vi "FPGA Top - Packet TX Only.vi"() -> ()   [LabVIEW 2017, in "My Network FPGA v1.lvlib"]
uses:
  My Network FPGA v1.lvlib
  <instrlib>/_niInstr/Network/Types/v1/MAC Address.ctl
  <instrlib>/_niInstr/Network/Types/v1/IPv4 Address.ctl
  <instrlib>/_niInstr/Network/Ethernet/MAC/CLIP/v1/Resources.ctl
  <vilib>/Platform/TimedLoop/XDataNode/timing_clust.ctl
  <vilib>/Platform/TimedLoop/XDataNode/nitl_modes.ctl
  <vilib>/Platform/TimedLoop/XDataNode/wakeup.ctl
  <vilib>/rvi/Emulation/niFpgaGetClockAttributes.vi
  <vilib>/rvi/Emulation/niFpgaSctlEmulationGetInTimedLoop.vi
  <vilib>/rvi/Emulation/niFpgaEmulationReportErrorSimple.vi
  <vilib>/rvi/DataTransferAndStorage/Container/Common/niFpgaContainerGetUniqueNameForEmu.vi
  <vilib>/rvi/DataTransferAndStorage/Container/Common/niFpgaContainerSetEmuInfo.vi
  <vilib>/rvi/eio/common/nirviEmuReportErrorAndStop.vi
  <vilib>/rvi/Emulation/niFpgaProcessEmulError.vi
  <vilib>/rvi/DataTransferAndStorage/Container/Common/niFpgaContainerExecOnDevCompGetState.vi
  <vilib>/rvi/Emulation/niFpgaEmulationIsFPGAContextNoSignature.vi
  <vilib>/rvi/errors/niFpgaSetErrorForExecOnDevCompSimple.vi
  <vilib>/rvi/FIFO/Fifo_Resource/nirvififoEmulationSetSize.vi
  <vilib>/rvi/FIFO/Fifo_Resource/nirviFifoEmulationQueueMgr.vi
  <instcachedir>/0/nirviFifoEmulationQueueMgr_E5CAEC123FF24DC58D834DCA3CDAA9B5.lvgen/nirviFifoEmulationQueueMgr_E5CAEC123FF24DC58D834DCA3CDAA9B5_003.vi
  <vilib>/rvi/FIFO/Fifo_Resource/nirvififoEmulationDetermineInputValidOut.vi
  <vilib>/rvi/FIFO/Fifo_Resource/nirvififoEmulationCreateLock.vi
  <vilib>/rvi/FIFO/Fifo_Resource/nirvififoEmulationObtainLock.vi
  <vilib>/rvi/FIFO/Fifo_Resource/nirvififoEmulationReleaseLock.vi
  <vilib>/rvi/occurrence/nirviWaitOnOccurrenceBase.vi
  <vilib>/rvi/errors/nirviReportUnexpectedCaseInternalError.vi
  <vilib>/rvi/errors/nirviReportUnexpectedCaseInternalError (U32).vi
  <vilib>/Utility/error.llb/Clear Errors.vi
  <vilib>/rvi/interface/RandomDataEmulation/niFpgaRandomDataHandleErrors.vi
  <vilib>/rvi/Emulation/niFpgaCriticalErrorInLSC.vi
  <vilib>/rvi/eio/common/nirviEmuTemplateMethod_errors.vi
  <vilib>/Platform/TimedLoop/XDataNode/XDataNode.xnode
  <vilib>/rvi/LocalResourceManager/LocalResourceManager.xnode
  <vilib>/rvi/DataTransferAndStorage/Container/XNode/niFpgaContainer.xnode
  <vilib>/rvi/FIFO/Fifo_Resource/niFpgaFifoEmulationRefIn.vi
  <vilib>/eio/EIONode/EIONode.xnode
  <instrlib>/_niInstr/Network/Ethernet/MAC/CLIP/v1/niInstr Ethernet MAC - CLIP v1.lvclass
  <instrlib>/_niInstr/Network/Ethernet/MAC/Raw Stream/v1/niInstr Ethernet MAC Raw Stream v1.lvclass
  <vilib>/Platform/TimedLoop/XDataNode/XDNodeRunTimeDep.lvlib
  <instrlib>/_niInstr/Network/IPv4/UDP/FPGA/v1/niInstr IPv4 UDP FPGA v1.lvlib
  <instrlib>/_niInstr/Network/Types/v1/niInstr Network Types v1.lvlib
panel:
  in  "enable tx":bool=TRUE
  in  "max payload per frame":u16=1472
  in  "send packet":bool
  in  "udp payload length":u16=1024
  out "aBlockLockPort0":bool
  out "aBlockLockPort1":bool
  out "mgtrefclks_locked":bool
  out "mgtrefclks_valid":bool
  out "posc_complete":bool
  out "sPort0_Power_Good":bool
  out "sPort1_Power_Good":bool
  out "signal_detect_Port0":bool
  out "signal_detect_Port1":bool
  in  "UDP destination port":u16=35311
  in  "MAC destination address":T1=[255, 255, 255, 255, 255, 255] format="%.0x"
  in  "IPv4 destination address":T2=[255, 255, 255, 255]
  in  "UDP source port":u16
  in  "IPv4 source address":T2=[0, 0, 0, 0]
  in  "MAC source address":T1=[0, 128, 47, 0, 0, 1] format="%.0x"
  # "License Note\n\nThis example makes use of code under the LGPLv2 license in the Socketed CLIP to support 10 Gigabit Ethernet.  You may find the source and build instructions for this component in the CLIP directory."
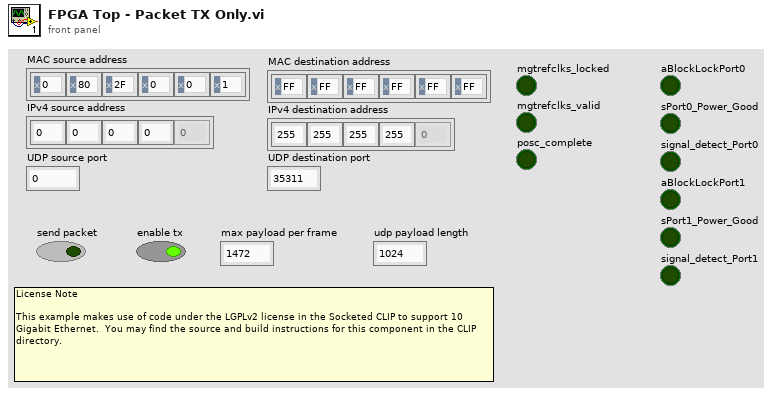
[diagram p1: front panel]
types:
  T1 = typedef "niInstr Network Types v1.lvlib/MAC Address.ctl" = u8[]
  T2 = typedef "niInstr Network Types v1.lvlib/IPv4 Address.ctl" = u8[]
  T3 = typedef "niInstr Ethernet MAC - CLIP v1.lvclass/Resources.ctl" = cluster{"RX":cluster{"TData":refnum<k21>, "TValid":refnum<k21>, "TKeep":refnum<k21>, "TLast":refnum<k21>, "TUser":refnum<k21>}, "TX":cluster{"TData":refnum<k21>, "TValid":refnum<k21>, "TKeep":refnum<k21>, "TLast":refnum<k21>, "TReady":refnum<k21>}, "Pause resources":cluster{"cPauseValuePort":refnum<k21>, "cPauseReqPort":refnum<k21>}, "MAC Clock":refnum<k21>}
  T4 = typedef "XDNodeRunTimeDep.lvlib/timing_clust.ctl" = cluster{"Expected End [f-1]":u64, "Actual End [f-1]":u64, "Finished Late? [f-1]":bool, "Expected End [i-1]":u64, "Actual End [i-1]":u64, "Finished Late? [i-1]":bool, "Expected Start [i]":u64, "Actual Start [i]":u64, "Expected Start [f]":u64, "Actual Start [f]":u64, "Source Name":string, "Structure Name":string, "Period":i64, "Deadline":i64, "Offset":i64, "Start":i64, "Priority":i32, "Timeout":i32, "Mode":T5, "Wakeup Reason":T6, "Error":errorcluster, "Source Type":string, "Secondary Source Type":string, "Global End Time":u64, "Global Start Time":u64, "Frame Duration":u64, "Iteration Duration":u64, "Assigned CPU":i32, "I/O Scan Engine Mode":u32}
  T5 = typedef "XDNodeRunTimeDep.lvlib/nitl_modes.ctl" = enum32{"No Change", "Process missed periods, maintain original phase", "Discard missed periods, maintain original phase", "Process missed periods, ignore original phase", "Discard missed periods, ignore original phase"}
  T6 = typedef "XDNodeRunTimeDep.lvlib/wakeup.ctl" = enum32{"Normal", "Aborted", "Asynchronous wakeup", "Timing source error", "Timed loop error", "Timeout"}
  T7 = cluster{"ready for input (payload data)":bool, "ready for input (start packet)":bool}
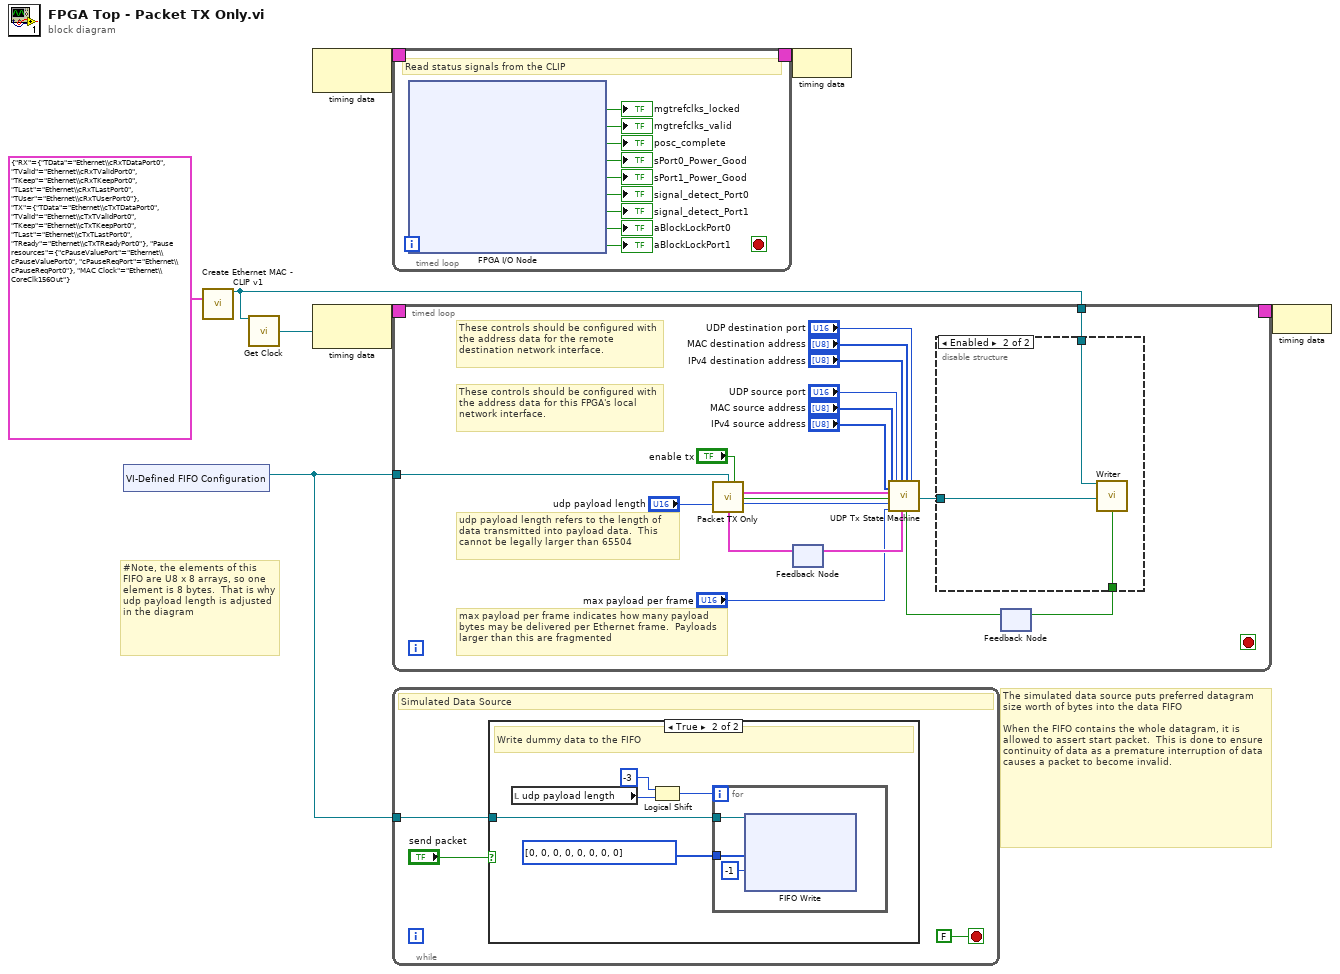
[diagram p0: block diagram]
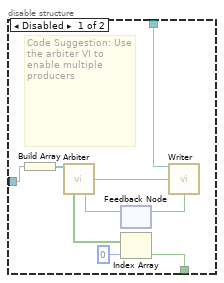
[diagram p3: hidden frame]
diagram:
  # "#Note, the elements of this FIFO are U8 x 8 arrays, so one element is 8 bytes.  That is why udp payload length is adjusted in the diagram"
  # "The simulated data source puts preferred datagram size worth of bytes into the data FIFO\n\nWhen the FIFO contains the whole datagram, it is allowed to assert start packet.  This is done to ensure continuity of data as a premature interruption of data causes a packet to become invalid."
  n1 = xnode "VI-Defined FIFO Configuration"() -> ("FIFO Out"=w4:refnum<k21>)
  n2 = call <instrlib>:"Create Ethernet MAC - CLIP v1.vi"("Ethernet AXI4-S Resources"=T3 {"RX"={"TData"="Ethernet\\cRxTDataPort0", "TValid"="Ethernet\\cRxTValidPort0", "TKeep"="Ethernet\\cRxTKeepPort0", "TLast"="Ethernet\\cRxTLastPort0", "TUser"="Ethernet\\cRxTUserPort0"}, "TX"={"TData"="Ethernet\\cTxTDataPort0", "TValid"="Ethernet\\cTxTValidPort0", "TKeep"="Ethernet\\cTxTKeepPort0", "TLast"="Ethernet\\cTxTLastPort0", "TReady"="Ethernet\\cTxTReadyPort0"}, "Pause resources"={"cPauseValuePort"="Ethernet\\cPauseValuePort0", "cPauseReqPort"="Ethernet\\cPauseReqPort0"}, "MAC Clock"="Ethernet\\CoreClk156Out"}) -> ("niInstr Ethernet MAC - CLIP v1.lvclass out"=w5:refnum<class "niInstr Ethernet MAC - CLIP v1.lvclass">)  [unwired: 14 in]
  n3 = call-dynamic "Get Clock.vi"("niInstr Ethernet MAC - CLIP v1.lvclass"=w5) -> ("MAC Clock"=w1:refnum<k21>)  [unwired: 14 in]
  n4 = node-c288() -> (w3:T4)  [unwired: 1 in]
  n5 = node-c288(w1) -> (w7:T4)
  n6 = timed-loop {
    timing: w3 -> [_]
    timing-out: [_] -> w2
    stop <- _ stop-if-true
    # "Read status signals from the CLIP"
    n7 = xnode "FPGA I/O Node"() -> ("Ethernet\\MgtRefClks_Locked"=→"mgtrefclks_locked":bool, "Ethernet\\MgtRefClks_Valid"=→"mgtrefclks_valid":bool, "Ethernet\\POSC_Complete"=→"posc_complete":bool, "Ethernet\\sPort0_Power_Good"=→"sPort0_Power_Good":bool, "Ethernet\\sPort1_Power_Good"=→"sPort1_Power_Good":bool, "Ethernet\\signal_detect_Port0"=→"signal_detect_Port0":bool, "Ethernet\\signal_detect_Port1"=→"signal_detect_Port1":bool, "Ethernet\\aBlockLockPort0"=→"aBlockLockPort0":bool, "Ethernet\\aBlockLockPort1"=→"aBlockLockPort1":bool)  [unwired: 9 in, 9 out]
  }
  n8 = timed-loop {
    timing: w7 -> [_]
    timing-out: [_] -> w6
    tunnel: w5 -> [w38]
    tunnel: w4 -> [w25]
    stop <- _ stop-if-true
    # "udp payload length refers to the length of data transmitted into payload data.  This cannot be legally larger than 65504"
    # "max payload per frame indicates how many payload bytes may be delivered per Ethernet frame.  Payloads larger than this are fragmented"
    # "These controls should be configured with the address data for this FPGA's local network interface."
    # "These controls should be configured with the address data for the remote destination network interface."
    n9 = feedback #1() -> (w24:T7)  [unwired: 1 in]
    n10 = call "Packet TX Only.vi"("payload fifo"=w25, "enable tx"="enable tx", "udp payload length"="udp payload length", "ready for input"=w24) -> ("payload data"=w21:cluster{"Element":u8[], "Output Valid":bool}, "start packet"=w22:bool, "payload length"=w23:u16)  [unwired: 9 in]
    n11 = feedback #2() -> (w34:bool)  [unwired: 1 in]
    n12 = call <instrlib>:"UDP Tx State Machine.vi"("MAC source address"="MAC source address", "IPv4 source address"="IPv4 source address", "payload data"=w21, "start packet"=w22, "payload length"=w23, "max payload per frame"="max payload per frame", "UDP source port"="UDP source port", "IPv4 destination address"="IPv4 destination address", "MAC destination address"="MAC destination address", "ready for output"=w34, "UDP destination port"="UDP destination port") -> ("ready for input"=w35:T7, "niInstr Ethernet MAC Raw Stream v1 out"=w37:refnum<class "niInstr Ethernet MAC Raw Stream v1.lvclass">)  [unwired: 7 in]
    n13 = feedback-in #1(w35) -> ()
    n14 = disable-structure shown="Enabled" {
      disable-tunnel: w38 -> [w43 w48]
      disable-tunnel: w37 -> [w41 w49]
      disable-tunnel: [w40 w50] -> w36
      frame Disabled {
        # "Code Suggestion: Use the arbiter VI to enable multiple producers"
        n15 = Build Array(w41) -> (w42:refnum<class "niInstr Ethernet MAC Raw Stream v1.lvclass">[])
        n16 = feedback #3() -> (w45:bool)  [unwired: 1 in]
        n17 = call <instrlib>:"Arbiter.vi"("inbound packet streams"=w42, "ready for output"=w45) -> ("element"=w47:refnum<class "niInstr Ethernet MAC Raw Stream v1.lvclass">, "ready for input"=w46:bool[])  [unwired: 12 in]
        n18 = Index Array(array=w46, index=0) -> (element=w40:bool)
        n19 = call-dynamic "Writer.vi"("niInstr Ethernet MAC v1.lvclass"=w43, "niInstr Ethernet MAC Raw Stream v1.lvclass"=w47) -> ("ready for input?"=w44:bool)  [unwired: 12 in, 1 out]
        n20 = feedback-in #3(w44) -> ()
      }
      frame Enabled {
        n21 = call-dynamic "Writer.vi"("niInstr Ethernet MAC v1.lvclass"=w48, "niInstr Ethernet MAC Raw Stream v1.lvclass"=w49) -> ("ready for input?"=w50:bool)  [unwired: 12 in, 1 out]
      }
    }
    n22 = feedback-in #2(w36) -> ()
  }
  n23 = while {
    tunnel: w4 -> [w54]
    stop <- FALSE stop-if-true
    # "Simulated Data Source"
    n24 = case shown="True" "send packet" {
      tunnel: w54 -> [_ w57]
      frame False {
      }
      frame True {
        # "Write dummy data to the FIFO"
        n25 = local read "udp payload length"() -> (w59:u16)
        n26 = Logical Shift(y=i16 -3, x=w59) -> (x << y=w58:u16)
        n27 = for {
          N: w58 -> [_]
          tunnel: w57 -> [w63]
          tunnel: u8[] [0, 0, 0, 0, 0, 0, 0, 0] ("Element") -> [w62]
          n28 = xnode "FIFO Write"("Element"=w62, "Timeout"=-1, "FIFO In"=w63) -> ()  [unwired: 2 out]
        }
      }
    }
  }
  n29 = node-c288(w2) -> ()
  n30 = node-c288(w6) -> ()
